vi "Create Banking Statement from CSV.vi"(8 "error in (no error)":errorcluster, 11 "CSV Entries":string[](array[string])) -> (0 "error out":errorcluster, 3 "Statement.lvclass":refnum<class "Statement.lvclass">)   [LabVIEW 2018, in "Statement.lvclass"]
uses:
  Statement/Statement.lvclass
  Statement/Statement.lvclass/Statement.ctl
  Banking Record/Banking Transaction.lvclass
  C:/Users/jtipps/Documents/Filthy-Lucre-Budgetizer/source/support/classes/Transaction/Transaction.lvclass
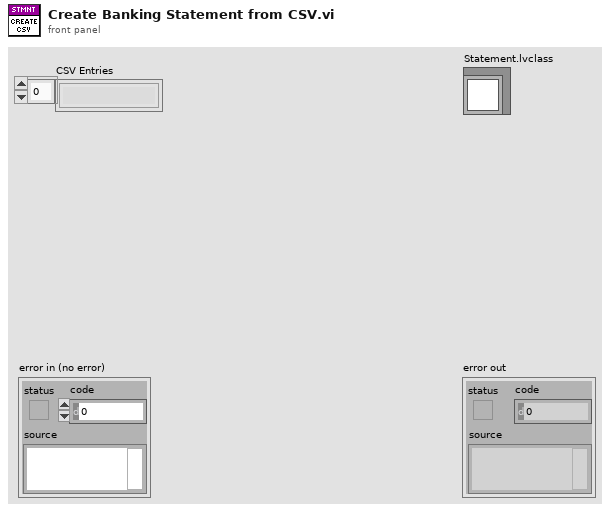
[diagram p1: front panel]
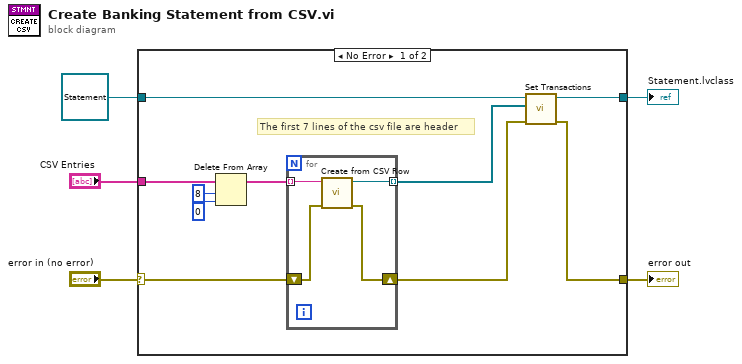
[diagram p0: block diagram]
diagram:
  n1 = case shown="No Error" "error in (no error)" {
    selector: "error in (no error)" -> [w15 w21]
    tunnel: [w11 w21] -> w4
    tunnel: refnum<class "Statement.lvclass"> refnum ("Statement.lvclass") -> [w14 w20]
    tunnel: [w13 w20] -> w3
    tunnel: "CSV Entries" -> [w7 _]
    frame No Error {
      # "The first 7 lines of the csv file are header"
      n2 = Delete From Array(array=w7, length=8, index=0) -> (array with subset deleted=w6:string[])  [unwired: 1 out]
      n3 = for {
        tunnel: w6 -> [w18] mode=indexing
        tunnel: [w19] -> w10 mode=indexing
        shift-right: [w16] -> w12
        shift-left: w15 -> [w17]
        n4 = call "Create from CSV Row.vi"("error in (no error)"=w17, "CSV Row"=w18) -> ("error out"=w16:errorcluster, "Banking Record"=w19:refnum<class "Banking Transaction.lvclass">)  [unwired: 8 in]
      }
      n5 = call "Set Transactions.vi"("error in (no error)"=w12, "Transactions"=w10, "Statement in"=w14) -> ("error out"=w11:errorcluster, "Statement out"=w13:refnum<class "Statement.lvclass">)  [unwired: 7 in]
    }
    frame Error {
    }
  }
  "error out" <- w4
  "Statement.lvclass" <- w3
